vi "FRCts20_WebMethods_Notifications_GET.vi"(7 "httpRequestID":u32) -> ()   [LabVIEW 2013, in "FRCts20_WebMethods.lvlib"]
uses:
  FRCts20_WebMethods.lvlib
  ESP Engine/source/VI Source/FRCts20_EspEngine.lvlib
  Backend/source/VI Source/FRCts20_Backend_API/FRCts20_Backend_API.lvlib
  Backend/source/VI Source/FRCts20_Backend_API/FRCts20_Backend_API_EventRoot.vi
  Backend/source/VI Source/FRCts20_Backend_API/FRCts20_Backend_API_Command_EventRoot.ctl
  Backend/source/VI Source/FRCts20_Backend_API/FRCts20_Backend_API_EventRoot.ctl
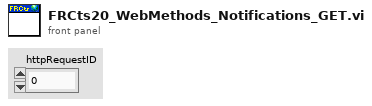
[diagram p1: front panel]
types:
  T1 = typedef "FRCts20_Backend_API.lvlib/FRCts20_Backend_API_EventRoot.ctl" = cluster{"Event":cluster{"Event Index":u32, "Event Name":string, "Start Time":timestamp, "End Time":timestamp, "OpenIssues":u8, "IsLive":bool}[], "APIReturn":string}
  T2 = typedef "FRCts20_Backend_API.lvlib/FRCts20_Backend_API_Command_EventRoot.ctl" = string
  T3 = typedef "FRCts20_EspEngine.lvlib/FRCts20_EspEngine_SearchBrowser.ctl" = cluster{"Event":cluster{"Event Index":u32, "Event Name":string, "Start Time":timestamp, "End Time":timestamp, "OpenIssues":u8, "IsLive":bool}[], "select-choice-software":string, "select-choice-location":string}
  T4 = typedef "FRCts20_EspEngine.lvlib/FRCts20_EspEngine_Universe.ctl" = cluster{"TeamsListLength":i16, "Teams":T5[], "LiveEventListLength":i16, "LiveEvents":T11[], "NonLiveEventListLength":i16, "NonLiveEvents":T11[], "OpenIssueCount":i16, "NotFoundStatus":bool}
  T5 = typedef "FRCts20_EspEngine.lvlib/FRCts20_EspEngine_Team.ctl" = cluster{"Team":T6, "RequestListLength":i16, "Requests":T9[]}
  T6 = typedef "FRCts20_WebMethods.lvlib/FRCts20_WebMethods_ctl_singleTeam.ctl" = cluster{"Events":string[], "Robot Name":string, "Kinect":bool, "Vision":bool, "Can":bool, "Tags":string, "Avatar URL":string, "Team":T7, "SWType":T8}
  T7 = typedef "FRCts20_WebMethods.lvlib/FRCts20_WebMethods_ctl_teamIdentifier.ctl" = cluster{"Team Nickname":string, "Team Number ":u32, "UniqueId":u32}
  T8 = typedef "FRCts20_Backend_API.lvlib/FRCts20_Backend_API_SW.ctl" = string
  T9 = typedef "FRCts20_WebMethods.lvlib/FRCts20_WebMethods_ctl_request.ctl" = cluster{"Event":string, "Description":string, "Status":T10, "Open Date":string, "Last Update":string, "Close Date":string, "UniqueId":i32, "Team":cluster{"Team Nickname":string, "Team Number ":i32, "UniqueId":i32}, "Comments":cluster{"Request Number":dbl, "Text":string, "Author":string, "IsSolution":bool, "Team":cluster{"Team Nickname":string, "Team Identifier ":dbl}, "UniqueId":i32}[]}
  T10 = typedef "FRCts20_Backend_API.lvlib/FRCts20_Backend_API_Status.ctl" = enum16{"Open", "In Work", "Closed"}
  T11 = typedef "FRCts20_EspEngine.lvlib/FRCts20_EspEngine_Event.ctl" = cluster{"Single Event":T12, "EventOpenIssueCount":i16, "Requests":cluster{"RequestId":i32, "Request Description":string, "Team Number":i32}[], "ClosedRequests":cluster{"RequestId":i32, "Request Description":string, "Team Number":i32}[], "NotFoundStatus":bool}
  T12 = typedef "FRCts20_WebMethods.lvlib/FRCts20_WebMethods_ctl_singleEvent.ctl" = cluster{"Team":T7[], "Issue Count":i32, "Location":string, "Start Date ":timestamp}
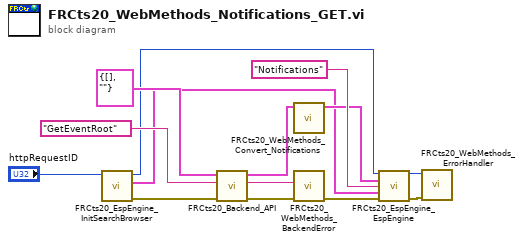
[diagram p0: block diagram]
diagram:
  n1 = call "FRCts20_EspEngine_InitSearchBrowser.vi"("httpRequestID"="httpRequestID") -> ("error out"=w4:errorcluster, "SearchBrowser"=w3:T3, "httpRequestID out"=w1:u32)  [unwired: 8 in]
  n2 = call-poly "FRCts20_Backend_API.vi"("error in (no error)"=w4, "Message"=T2 "GetEventRoot", "EventRoot In"=T1 {"Event"=[], "APIReturn"=""}) -> ("error out"=w9:errorcluster, "Status"=w8:string, "EventRoot Out"=w6:T1)  [unwired: 6 in]
  n3 = call "FRCts20_WebMethods_Convert_Notifications.vi"("EventRoot Out"=w6) -> ("Universe"=w5:T4)  [unwired: 9 in, 1 out]
  n4 = call "FRCts20_WebMethods_BackendError.vi"("error in (no error)"=w9, "Status"=w8) -> ("error out"=w7:errorcluster)  [unwired: 8 in, 1 out]
  n5 = call "FRCts20_EspEngine_EspEngine.vi"("httpRequestID"=w1, "Cluster"=w5, "Page"="Notifications", "SearchBrowser"=w3, "error in (no error)"=w7) -> ("httpRequestID out"=w13:u32, "error out"=w14:errorcluster)  [unwired: 9 in]
  n6 = call "FRCts20_WebMethods_ErrorHandler.vi"("error in"=w14, "httpRequestID"=w13) -> ()  [unwired: 9 in, 1 out]
